vi "Running.vi"(0 "DashboardServer in":refnum<class "Dashboard Server.lvclass">, 5 "error in (no error)":errorcluster) -> (14 "DashboardServer out":refnum<class "Dashboard Server.lvclass">, 15 "running":bool, 19 "error out":errorcluster)   [LabVIEW 2016, in "Dashboard Server.lvclass"]
uses:
  Dashboard Server.lvclass
panel:
  out "returnStatus":string
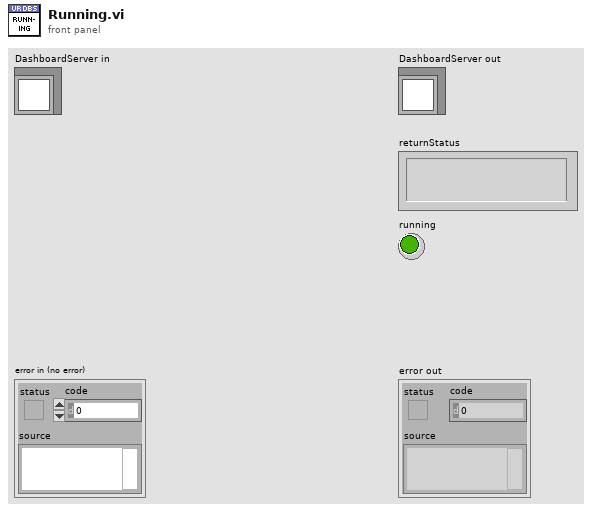
[diagram p1: front panel]
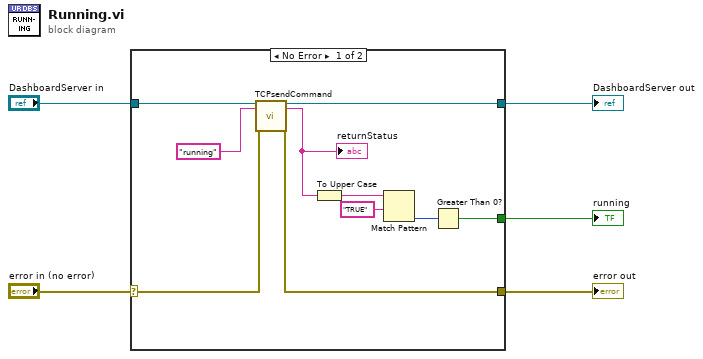
[diagram p0: block diagram]
diagram:
  n1 = case shown="No Error" "error in (no error)" {
    selector: "error in (no error)" -> [w13 w17]
    tunnel: [w12 w17] -> w4
    tunnel: [w14 w16] -> w2
    tunnel: "DashboardServer in" -> [w15 w16]
    tunnel: [w6 _] -> w1
    frame No Error {
      n2 = call-dynamic "TCPsendCommand.vi"("DashboardServer in"=w15, "command"="running", "error in (no error)"=w13) -> ("DashboardServer out"=w14:refnum<class "Dashboard Server.lvclass">, "returnStatus"=w10:string, "error out"=w12:errorcluster)  [unwired: 13 in, 1 out]
      "returnStatus" <- w10
      n3 = To Upper Case(1:w10) -> (0:w9:string)
      n4 = Match Pattern(string=w9, regular expression="TRUE") -> (offset past match=w7:i32)  [unwired: 1 in, 3 out]
      n5 = Greater Than 0?(x=w7) -> (x > 0?=w6:bool)
    }
    frame Error {
    }
  }
  "error out" <- w4
  "DashboardServer out" <- w2
  "running" <- w1
